vi "log_write.vi"(0 "type":string, 4 "neirong":string, 6 "ip_add":string, 8 "datetime":string, 9 "action":string, 10 "yw":string, 11 "user":string) -> (3 "error":errorcluster caption="error out 2")   [LabVIEW 2017, in "Lib_code.lvlib"]
uses:
  Lib_code.lvlib
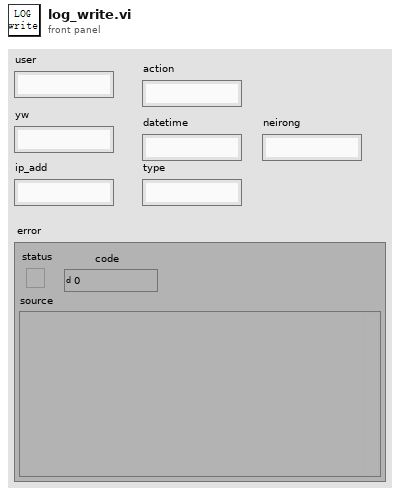
[diagram p1: front panel]
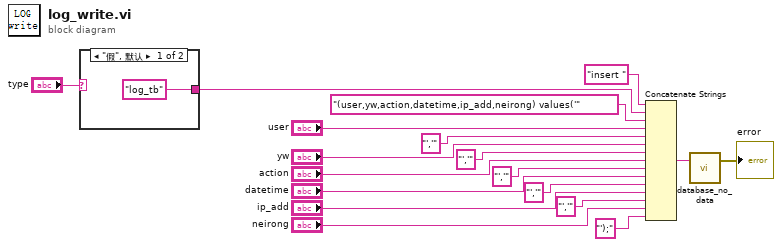
[diagram p0: block diagram]
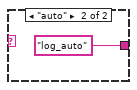
[diagram p2: hidden frame]
diagram:
  n1 = case shown="\"假\", 默认" "type" {
    tunnel: ["log_tb" "log_auto"] -> w2
    frame "假", Default {
    }
    frame "auto" {
    }
  }
  n2 = Concatenate Strings("insert " ("格式字符串"), w2, "(user,yw,action,datetime,ip_add,neirong) values('" ("格式字符串"), "user", "','" ("字符串"), "yw", "','" ("字符串"), "action", "','" ("字符串"), "datetime", "','" ("字符串"), "ip_add", "','" ("字符串"), "neirong", "');" ("字符串")) -> (w18:string)
  n3 = call "database_no_data.vi"("input"=w18) -> ("error"=→"error":errorcluster)  [unwired: 2 in]
